vi "P7.vi"() -> ()   [LabVIEW 2019]
panel:
  out "moving average":dbl
  out "previous result":dbl
  in  "stop":bool
  out "random number":dbl
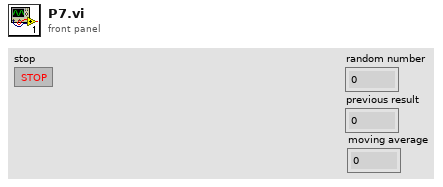
[diagram p1: front panel]
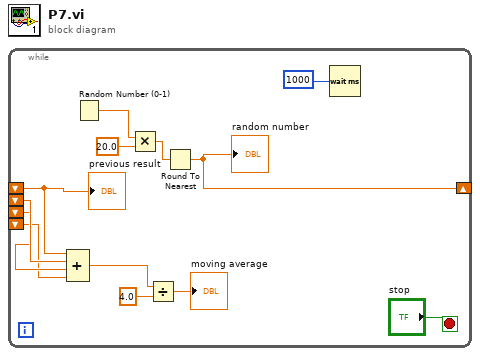
[diagram p0: block diagram]
diagram:
  n1 = while {
    shift-right: [w8] -> _
    shift-left: _ -> [w5]
    shift-left: _ -> [w4]
    shift-left: _ -> [w3]
    shift-left: _ -> [w2]
    stop <- "stop" stop-if-true
    n2 = Compound Arithmetic op=ADD(w5, w4, w3, w2) -> (w6:dbl)
    n3 = Random Number (0-1)() -> (number: 0 to 1=w12:dbl)
    n4 = Multiply(x=w12, y=20.0) -> (x*y=w11:dbl)
    n5 = Divide(x=w6, y=4.0) -> (x/y=→"moving average":dbl)
    n6 = Round To Nearest(number=w11) -> (nearest integer value=w8:dbl)
    "random number" <- w8
    n7 = Wait (ms)(milliseconds to wait=u32 1000) -> ()  [unwired: 1 out]
    "previous result" <- w5
  }
